vi "Replace Element of Sections by Name.vi"(8 "error in (no error)":errorcluster, 9 "Section":refnum<class "Section.lvclass">, 10 "Section Name":string, 11 "Configuration in":refnum<class "Configuration.lvclass">) -> (0 "error out":errorcluster, 1 "Found?":bool, 3 "Configuration out":refnum<class "Configuration.lvclass">)   [LabVIEW 2014, in "Configuration.lvlib" / "Configuration.lvclass"]
doc: "Replace section by name in class private data."
uses:
  Configuration.lvclass
  Section/Section.lvclass
  Configuration.lvclass/Configuration.ctl
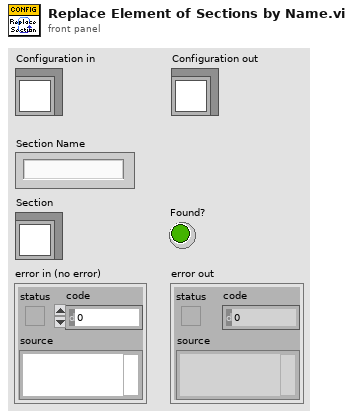
[diagram p1: front panel]
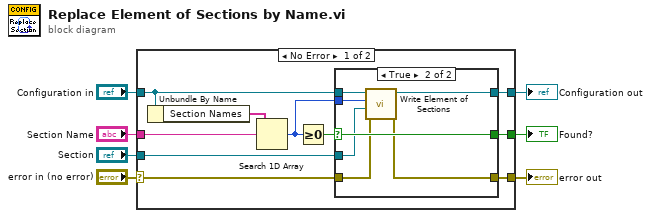
[diagram p0: block diagram]
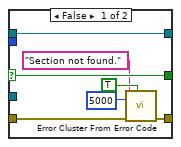
[diagram p2: hidden frame]
diagram:
  n1 = case shown="No Error" "error in (no error)" {
    selector: "error in (no error)" -> [w8 w32]
    tunnel: [w9 w32] -> w6
    tunnel: [w13 w33] -> w4
    tunnel: "Configuration in" -> [w14 w33]
    tunnel: "Section Name" -> [w17 _]
    tunnel: [w11 _] -> w2
    tunnel: "Section" -> [w15 _]
    frame No Error {
      n2 = Unbundle By Name(w14) -> ("Section Names"=w10:string[])
      n3 = Search 1D Array(1D array=w10, element=w17) -> (index of element=w16:i32)  [unwired: 1 in]
      n4 = Greater Or Equal To 0?(x=w16) -> (x >= 0?=w12:bool)
      n5 = case shown="True" w12 {
        selector: w12 -> [w24 w31]
        tunnel: w16 -> [_ w27]
        tunnel: w15 -> [_ w26]
        tunnel: w14 -> [w23 w30]
        tunnel: [w23 w25] -> w13
        tunnel: [w24 w31] -> w11
        tunnel: [w21 w28] -> w9
        tunnel: w8 -> [w22 w29]
        frame False {
          n6 = call <vilib>:"Error Cluster From Error Code.vi"("show call chain? (False)"=TRUE, "error in (no error)"=w22, "error message (\"\")"="Section not found." ("error message (\"\")"), "error code (0)"=5000) -> ("error out"=w21:errorcluster)  [unwired: 5 in]
        }
        frame True {
          n7 = call "Write Element of Sections.vi"("error in (no error)"=w29, "Section"=w26, "index"=w27, "Configuration in"=w30) -> ("error out"=w28:errorcluster, "Configuration out"=w25:refnum<class "Configuration.lvclass">)  [unwired: 6 in]
        }
      }
    }
    frame Error {
    }
  }
  "error out" <- w6
  "Configuration out" <- w4
  "Found?" <- w2
